vi "Syringe Pressure to Cylinder Setpoint.vi"(8 "error in (no error)":errorcluster, 10 "Syringe Pressure":dbl, 11 "Cylinder in":refnum<class "Cylinder.lvclass">) -> (0 "error out":errorcluster, 2 "Cylinder Setpoint":dbl, 3 "Cylinder out":refnum<class "Cylinder.lvclass">)   [LabVIEW 2015, in "cRIO-Carbondioxide.lvlib" / "CO2-Actor.lvlib" / "Cylinder.lvclass"]
uses:
  Cylinder.lvclass
  Cylinder.lvclass/Cylinder.ctl
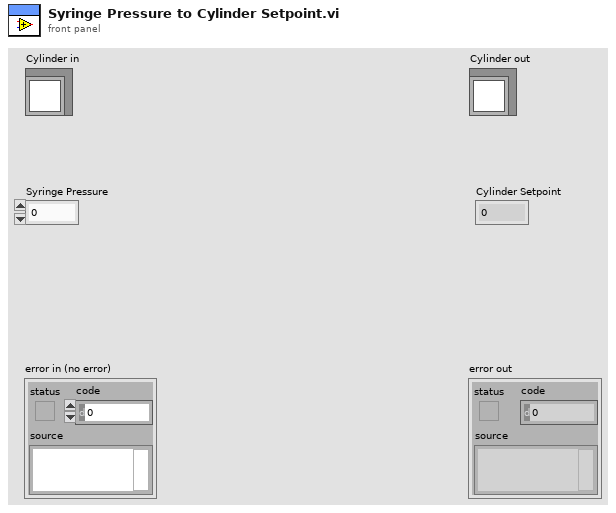
[diagram p1: front panel]
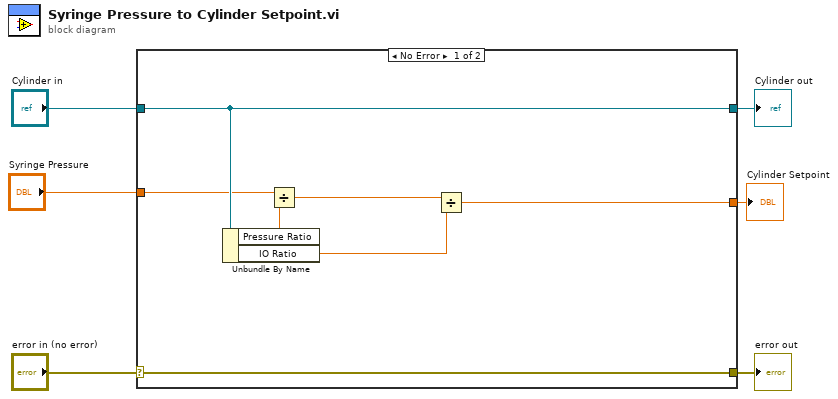
[diagram p0: block diagram]
diagram:
  n1 = case shown="No Error" "error in (no error)" {
    selector: "error in (no error)" -> [w13 w15]
    tunnel: [w13 w15] -> w5
    tunnel: [w12 w14] -> w3
    tunnel: "Cylinder in" -> [w12 w14]
    tunnel: "Syringe Pressure" -> [w11 _]
    tunnel: [w7 _] -> w1
    frame No Error {
      n2 = Unbundle By Name(w12) -> ("Pressure Ratio"=w10:dbl, "IO Ratio"=w8:dbl)
      n3 = Divide(x=w11, y=w10) -> (x/y=w9:dbl)
      n4 = Divide(x=w9, y=w8) -> (x/y=w7:dbl)
    }
    frame Error {
    }
  }
  "error out" <- w5
  "Cylinder out" <- w3
  "Cylinder Setpoint" <- w1
